vi "Define Default Prefix.vi"(8 "error in":errorcluster, 11 "Thermocouple Channel in":refnum<class "Thermocouple Channel.lvclass">) -> (0 "error out":errorcluster, 3 "Thermocouple Channel out":refnum<class "Thermocouple Channel.lvclass">)   [LabVIEW 2017, in "Scan Engine Scripting.lvlib" / "Thermocouple Channel.lvclass"]
uses:
  Thermocouple Channel.lvclass
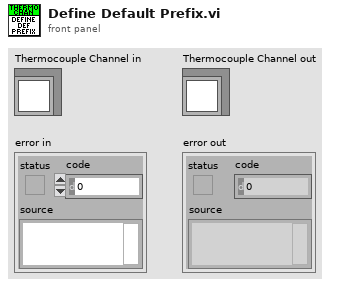
[diagram p1: front panel]
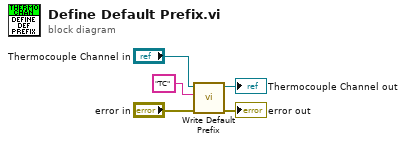
[diagram p0: block diagram]
diagram:
  n1 = call-dynamic "Write Default Prefix.vi"("error in"="error in", "default prefix"="TC", "channel in"="Thermocouple Channel in") -> ("error out"=→"error out":errorcluster, "channel out"=→"Thermocouple Channel out":refnum<class "Thermocouple Channel.lvclass">)  [unwired: 7 in]
